vi "Get Keywords.vi"(8 "error in (no error)":errorcluster, 11 "Boolean Functions in":refnum<class "Boolean Functions.lvclass">) -> (0 "error out":errorcluster, 2 "Keywords":string[](array[string]), 3 "Boolean Functions out":refnum<class "Boolean Functions.lvclass">)   [LabVIEW 2019, in "Boolean Functions.lvclass"]
uses:
  Boolean Functions.lvclass
  functionsbase/functionbase.lvclass
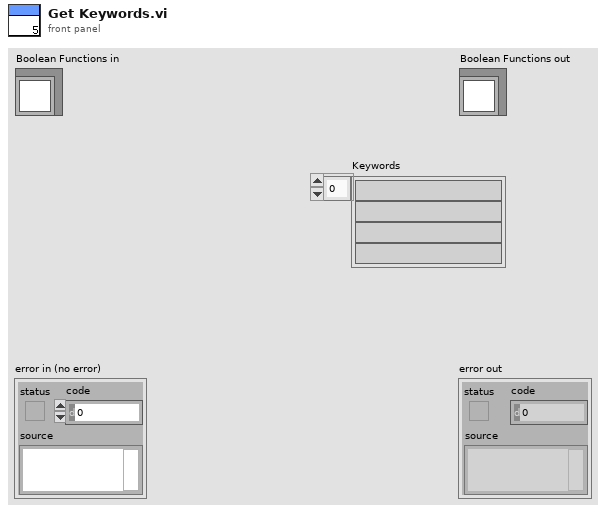
[diagram p1: front panel]
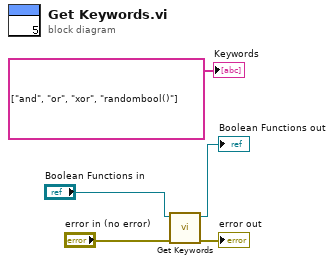
[diagram p0: block diagram]
diagram:
  n1 = call-parent "Get Keywords.vi"("error in (no error)"="error in (no error)", "functionbase in"="Boolean Functions in") -> ("error out"=→"error out":errorcluster, "functionbase out"=→"Boolean Functions out":refnum<class "Boolean Functions.lvclass">)  [unwired: 7 in, 1 out]
  "Keywords" <- string[] ["and", "or", "xor", "randombool()"] ("Keywords")
